vi "define.vi"(8 "error in (no error)":errorcluster, 11 "TrajectoryDL120126ArbitraryLine2D in":refnum<class "TrajectoryDL120126ArbitraryLine2D.lvclass">) -> (0 "error out":errorcluster, 3 "TrajectoryDL120126ArbitraryLine2D out":refnum<class "TrajectoryDL120126ArbitraryLine2D.lvclass">)   [LabVIEW 2010, in "TrajectoryDL120126ArbitraryLine2D.lvclass"]
doc: "modal dialog on which the user can set the trajectory parameters"
uses:
  TrajectoryDL120126ArbitraryLine2D.lvclass
  common/classes/SpaceVector/SpaceVector/SpaceVector.lvclass
  segment_cluster.ctl
panel:
  out "i":i32
  out "j":i32
  out "XY Graph":cluster{dbl, dbl}[](graph)
  in  "kappa":i32
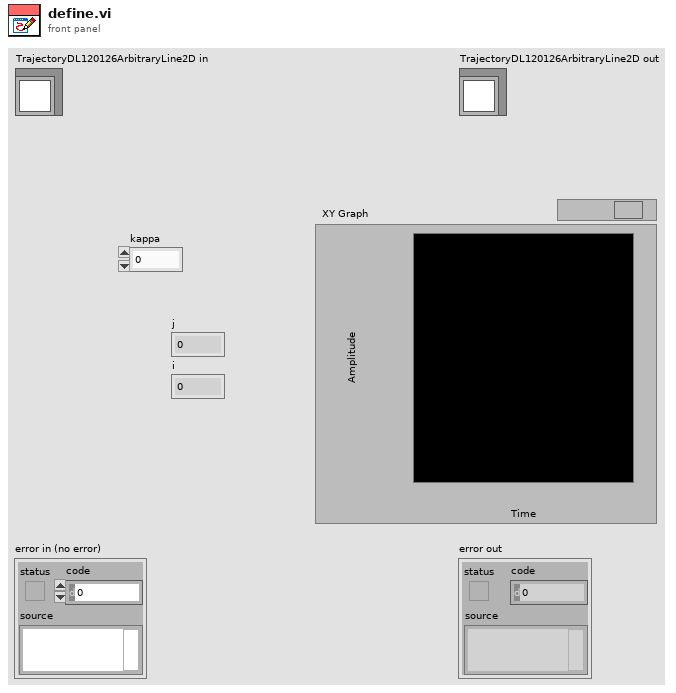
[diagram p1: front panel]
types:
  T1 = typedef "TrajectoryDL120126ArbitraryLine2D.lvclass/segment_cluster.ctl" = cluster{"points":refnum<class "SpaceVector.lvclass">[]}
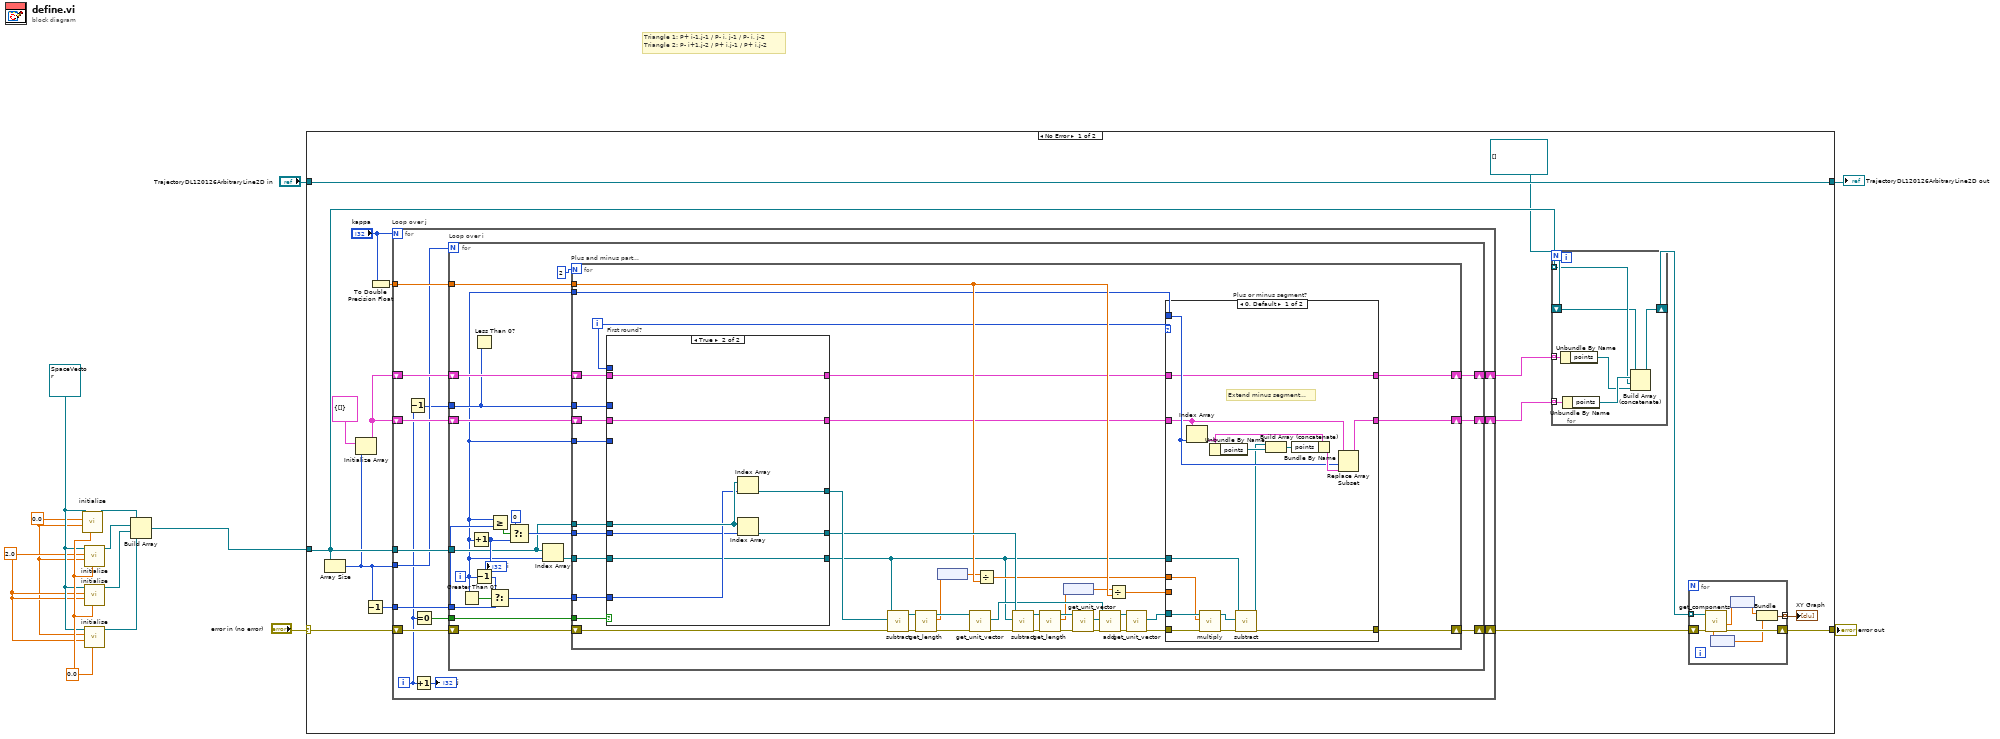
[diagram p0: block diagram]
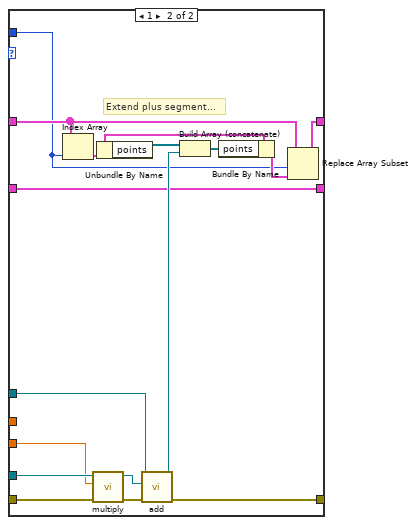
[diagram p2: hidden frame]
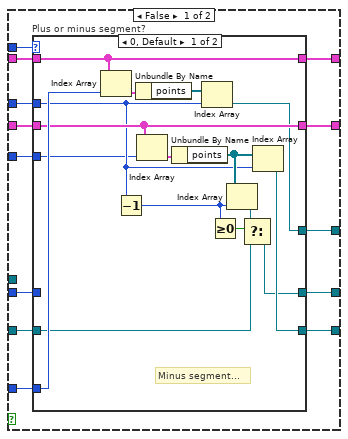
[diagram p3: hidden frame]
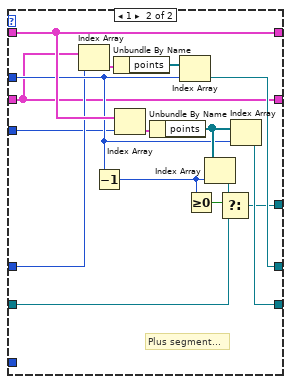
[diagram p4: hidden frame]
diagram:
  w7 = dbl[unit] 2.0 ("x")
  w6 = dbl[unit] 0.0 ("x")
  w9 = dbl[unit] 0.0 ("z")
  w8 = refnum<class "SpaceVector.lvclass"> refnum ("SpaceVector.lvclass")
  # "Triangle 1: P+ i-1,j-1 / P- i, j-1 / P- i, j-2\nTriangle 2: P- i+1,j-2 / P+ i,j-1 / P+ i,j-2"
  n1 = call "initialise.vi"("z"=w9, "y"=w6, "x"=w6, "SpaceVector in"=w8) -> ("SpaceVector out"=w5:refnum<class "SpaceVector.lvclass">)  [unwired: 6 in, 1 out]
  n2 = call "initialise.vi"("z"=w9, "y"=w6, "x"=w7, "SpaceVector in"=w8) -> ("SpaceVector out"=w4:refnum<class "SpaceVector.lvclass">)  [unwired: 6 in, 1 out]
  n3 = call "initialise.vi"("z"=w9, "y"=w7, "x"=w7, "SpaceVector in"=w8) -> ("SpaceVector out"=w3:refnum<class "SpaceVector.lvclass">)  [unwired: 6 in, 1 out]
  n4 = call "initialise.vi"("z"=w9, "y"=w7, "x"=w6, "SpaceVector in"=w8) -> ("SpaceVector out"=w2:refnum<class "SpaceVector.lvclass">)  [unwired: 6 in, 1 out]
  n5 = Build Array(w5, w4, w3, w2) -> (w1:refnum<class "SpaceVector.lvclass">[])
  n6 = case shown="No Error" "error in (no error)" {
    selector: "error in (no error)" -> [w28 w208]
    tunnel: "TrajectoryDL120126ArbitraryLine2D in" -> [w29 w209]
    tunnel: [w20 w208] -> w11
    tunnel: [w29 w209] -> w10
    tunnel: w1 -> [w24 _]
    frame No Error {
      n7 = Array Size(array=w24) -> (size(s)=w17:i32)
      n8 = Initialize Array(T1 {"points"=[]} ("segment"), w17) -> (w15:T1[])
      n9 = Decrement(x=w17) -> (x-1=w25:i32)
      n10 = To Double Precision Float(number="kappa") -> (double precision float=w26:dbl)
      n11 = for "Loop over j" {
        N: "kappa" -> [_]
        tunnel: w24 -> [w56]
        shift-right: [w57] -> w21
        shift-left: w28 -> [w58]
        shift-right: [w54] -> w23
        shift-left: w15 -> [w55]
        shift-right: [w52] -> w22
        shift-left: w15 -> [w53]
        tunnel: w26 -> [w51]
        tunnel: w17 -> [w49]
        tunnel: w25 -> [w50]
        i -> [w46]
        n12 = Decrement(x=w46) -> (x-1=w47:i32)
        n13 = Increment(x=w46) -> (x+1=→"j":i32)
        n14 = Equal To 0?(x=w46) -> (x = 0?=w45:bool)
        n15 = for "Loop over i" {
          N: w49 -> [_]
          shift-right: [w77] -> w57
          shift-left: w58 -> [w79]
          tunnel: w56 -> [w62]
          shift-right: [w75] -> w54
          shift-left: w55 -> [w68]
          shift-right: [w76] -> w52
          shift-left: w53 -> [w66]
          tunnel: w51 -> [w78]
          tunnel: w50 -> [w65]
          tunnel: w47 -> [w63]
          tunnel: w45 -> [w61]
          i -> [w59]
          n16 = Greater Than 0?(x=w59) -> (x > 0?=w74:bool)
          n17 = Increment(x=w59) -> (x+1=w69:i32)
          "i" <- w69
          n18 = Less Than 0?(x=w63) -> ()  [unwired: 1 out]
          n19 = Decrement(x=w59) -> (x-1=w73:i32)
          n20 = Select(t=w73, s=w74, f=w65) -> (s? t:f=w67:i32)
          n21 = Greater Or Equal?(x=w59, y=w65) -> (x >= y?=w72:bool)
          n22 = Select(t=0, s=w72, f=w69) -> (s? t:f=w71:i32)
          n23 = Index Array(array=w62, index=w59) -> (element=w64:refnum<class "SpaceVector.lvclass">)
          n24 = for "Plus and minus part..." {
            N: 2 -> [_]
            tunnel: w78 -> [w104]
            tunnel: w71 -> [w93]
            tunnel: w59 -> [w82]
            tunnel: w67 -> [w91]
            tunnel: w64 -> [w89]
            tunnel: w63 -> [w88]
            tunnel: w62 -> [w87]
            tunnel: w61 -> [w86]
            shift-right: [w94] -> w75
            shift-left: w68 -> [w92]
            shift-right: [w95] -> w76
            shift-left: w66 -> [w90]
            shift-right: [w96] -> w77
            shift-left: w79 -> [w120]
            tunnel: w59 -> [w80]
            i -> [w81]
            n25 = case "First round?" shown="True" w86 {
              tunnel: [w160 w203] -> w122
              tunnel: [w162 w204] -> w121
              tunnel: w93 -> [w158 w205]
              tunnel: w92 -> [w164 w201]
              tunnel: w91 -> [w167 w206]
              tunnel: w90 -> [w163 w200]
              tunnel: w89 -> [w166 w202]
              tunnel: w88 -> [w165 _]
              tunnel: w87 -> [_ w207]
              tunnel: [w161 w202] -> w85
              tunnel: [w156 w201] -> w84
              tunnel: [w155 w200] -> w83
              tunnel: w81 -> [w159 _]
              tunnel: w80 -> [w157 _]
              frame False {
                n26 = case "Plus or minus segment?" shown="0, Default" w159 {
                  tunnel: w167 -> [w176 _]
                  tunnel: w166 -> [w175 w191]
                  tunnel: w165 -> [w173 w190]
                  tunnel: w164 -> [w172 w199]
                  tunnel: w163 -> [w174 w184]
                  tunnel: [w169 w189] -> w162
                  tunnel: [w171 w188] -> w161
                  tunnel: [w168 w187] -> w160
                  tunnel: w158 -> [_ w186]
                  tunnel: w157 -> [w170 w185]
                  tunnel: [w172 w199] -> w156
                  tunnel: [w174 w184] -> w155
                  frame 0, Default {
                    # "Minus segment..."
                    n27 = Index Array(array=w172, index=w176) -> (element=w183:T1)
                    n28 = Decrement(x=w173) -> (x-1=w179:i32)
                    n29 = Unbundle By Name(w183) -> ("points"=w182:refnum<class "SpaceVector.lvclass">[])
                    n30 = Index Array(array=w174, index=w170) -> (element=w181:T1)
                    n31 = Unbundle By Name(w181) -> ("points"=w180:refnum<class "SpaceVector.lvclass">[])
                    n32 = Index Array(array=w182, index=w173) -> (element=w168:refnum<class "SpaceVector.lvclass">)
                    n33 = Greater Or Equal To 0?(x=w179) -> (x >= 0?=w178:bool)
                    n34 = Index Array(array=w180, index=w179) -> (element=w177:refnum<class "SpaceVector.lvclass">)
                    n35 = Select(t=w177, s=w178, f=w175) -> (s? t:f=w169:refnum<class "SpaceVector.lvclass">)
                    n36 = Index Array(array=w180, index=w173) -> (element=w171:refnum<class "SpaceVector.lvclass">)
                  }
                  frame 1 {
                    # "Plus segment..."
                    n37 = Index Array(array=w184, index=w186) -> (element=w198:T1)
                    n38 = Decrement(x=w190) -> (x-1=w194:i32)
                    n39 = Unbundle By Name(w198) -> ("points"=w197:refnum<class "SpaceVector.lvclass">[])
                    n40 = Index Array(array=w199, index=w185) -> (element=w196:T1)
                    n41 = Unbundle By Name(w196) -> ("points"=w195:refnum<class "SpaceVector.lvclass">[])
                    n42 = Index Array(array=w197, index=w190) -> (element=w189:refnum<class "SpaceVector.lvclass">)
                    n43 = Greater Or Equal To 0?(x=w194) -> (x >= 0?=w193:bool)
                    n44 = Index Array(array=w195, index=w194) -> (element=w192:refnum<class "SpaceVector.lvclass">)
                    n45 = Select(t=w192, s=w193, f=w191) -> (s? t:f=w187:refnum<class "SpaceVector.lvclass">)
                    n46 = Index Array(array=w195, index=w190) -> (element=w188:refnum<class "SpaceVector.lvclass">)
                  }
                }
              }
              frame True {
                n47 = Index Array(array=w207, index=w205) -> (element=w204:refnum<class "SpaceVector.lvclass">)
                n48 = Index Array(array=w207, index=w206) -> (element=w203:refnum<class "SpaceVector.lvclass">)
              }
            }
            n49 = call "subtract.vi"("error in (no error)"=w120, "subtrahend"=w122, "SpaceVector in"=w85) -> ("error out"=w112:errorcluster, "SpaceVector out"=w113:refnum<class "SpaceVector.lvclass">)  [unwired: 7 in]
            n50 = call "get_length.vi"("error in (no error)"=w112, "SpaceVector in"=w113) -> ("error out"=w111:errorcluster, "length"=w105:dbl[unit], "SpaceVector out"=w110:refnum<class "SpaceVector.lvclass">)  [unwired: 7 in]
            n51 = node(w105) -> (w101:dbl)
            n52 = call "get_unit_vector.vi"("error in (no error)"=w111, "SpaceVector in"=w110) -> ("error out"=w119:errorcluster, "unit vector"=w117:refnum<class "SpaceVector.lvclass">)  [unwired: 7 in, 1 out]
            n53 = Divide(x=w101, y=w104) -> (x/y=w102:dbl)
            n54 = call "subtract.vi"("error in (no error)"=w119, "subtrahend"=w85, "SpaceVector in"=w121) -> ("error out"=w107:errorcluster, "SpaceVector out"=w109:refnum<class "SpaceVector.lvclass">)  [unwired: 7 in]
            n55 = call "get_length.vi"("error in (no error)"=w107, "SpaceVector in"=w109) -> ("error out"=w106:errorcluster, "length"=w100:dbl[unit], "SpaceVector out"=w108:refnum<class "SpaceVector.lvclass">)  [unwired: 7 in]
            n56 = node(w100) -> (w99:dbl)
            n57 = call "get_unit_vector.vi"("error in (no error)"=w106, "SpaceVector in"=w108) -> ("error out"=w116:errorcluster, "unit vector"=w118:refnum<class "SpaceVector.lvclass">)  [unwired: 7 in, 1 out]
            n58 = call "add.vi"("error in (no error)"=w116, "vector to be added"=w118, "SpaceVector in"=w117) -> ("error out"=w114:errorcluster, "SpaceVector out"=w115:refnum<class "SpaceVector.lvclass">)  [unwired: 7 in]
            n59 = Divide(x=w99, y=w104) -> (x/y=w97:dbl)
            n60 = call "get_unit_vector.vi"("error in (no error)"=w114, "SpaceVector in"=w115) -> ("error out"=w103:errorcluster, "unit vector"=w98:refnum<class "SpaceVector.lvclass">)  [unwired: 7 in, 1 out]
            n61 = case "Plus or minus segment?" shown="0, Default" w81 {
              tunnel: w103 -> [w129 w139]
              tunnel: w102 -> [w125 _]
              tunnel: w98 -> [w126 w154]
              tunnel: w97 -> [_ w153]
              tunnel: [w127 w150] -> w96
              tunnel: [w133 w140] -> w95
              tunnel: [w131 w147] -> w94
              tunnel: w85 -> [w124 w143]
              tunnel: w84 -> [w131 w142]
              tunnel: w83 -> [w132 w140]
              tunnel: w82 -> [w134 w141]
              frame 0, Default {
                # "Extend minus segment..."
                n62 = Index Array(array=w132, index=w134) -> (element=w137:T1)
                n63 = call "multiply.vi"("error in (no error)"=w129, "factor"=w125, "SpaceVector in"=w126) -> ("error out"=w128:errorcluster, "SpaceVector out"=w130:refnum<class "SpaceVector.lvclass">)  [unwired: 7 in]
                n64 = Unbundle By Name(w137) -> ("points"=w138:refnum<class "SpaceVector.lvclass">[])
                n65 = call "subtract.vi"("error in (no error)"=w128, "subtrahend"=w130, "SpaceVector in"=w124) -> ("error out"=w127:errorcluster, "SpaceVector out"=w123:refnum<class "SpaceVector.lvclass">)  [unwired: 7 in]
                n66 = Build Array (concatenate)(w123, w138) -> (w136:refnum<class "SpaceVector.lvclass">[])
                n67 = Bundle By Name(cluster=w137, "points"=w136) -> (w135:T1)
                n68 = Replace Array Subset(array=w132, new element=w135, index=w134) -> (w133:T1[])
              }
              frame 1 {
                # "Extend plus segment..."
                n69 = Index Array(array=w142, index=w141) -> (element=w146:T1)
                n70 = call "multiply.vi"("error in (no error)"=w139, "factor"=w153, "SpaceVector in"=w154) -> ("error out"=w151:errorcluster, "SpaceVector out"=w152:refnum<class "SpaceVector.lvclass">)  [unwired: 7 in]
                n71 = Unbundle By Name(w146) -> ("points"=w145:refnum<class "SpaceVector.lvclass">[])
                n72 = call "add.vi"("error in (no error)"=w151, "vector to be added"=w152, "SpaceVector in"=w143) -> ("error out"=w150:errorcluster, "SpaceVector out"=w144:refnum<class "SpaceVector.lvclass">)  [unwired: 7 in]
                n73 = Build Array (concatenate)(w145, w144) -> (w148:refnum<class "SpaceVector.lvclass">[])
                n74 = Bundle By Name(cluster=w146, "points"=w148) -> (w149:T1)
                n75 = Replace Array Subset(array=w142, new element=w149, index=w141) -> (w147:T1[])
              }
            }
          }
        }
      }
      n76 = for {
        tunnel: w24 -> [w41] mode=indexing
        shift-right: [w38] -> w19
        shift-left: refnum<class "SpaceVector.lvclass">[] [] -> [w39]
        tunnel: w23 -> [w44] mode=indexing
        tunnel: w22 -> [w43] mode=indexing
        n77 = Unbundle By Name(w44) -> ("points"=w40:refnum<class "SpaceVector.lvclass">[])
        n78 = Unbundle By Name(w43) -> ("points"=w42:refnum<class "SpaceVector.lvclass">[])
        n79 = Build Array (concatenate)(w39, w42, w41, w40) -> (w38:refnum<class "SpaceVector.lvclass">[])
      }
      n80 = for {
        shift-right: [w35] -> w20
        shift-left: w21 -> [w36]
        tunnel: w19 -> [w37] mode=indexing
        tunnel: [w30] -> w18 mode=indexing
        n81 = call "get_components.vi"("error in (no error)"=w36, "SpaceVector in"=w37) -> ("error out"=w35:errorcluster, "x"=w33:dbl[unit], "y"=w34:dbl[unit])  [unwired: 4 in, 3 out]
        n82 = node(w34) -> (w31:dbl)
        n83 = node(w33) -> (w32:dbl)
        n84 = Bundle(w32, w31) -> (w30:cluster{dbl, dbl})  [unwired: 1 in]
      }
      "XY Graph" <- w18
    }
    frame Error {
    }
  }
  "error out" <- w11
  "TrajectoryDL120126ArbitraryLine2D out" <- w10
